vi "PH_BL-Master.set Instance remote controlled.vi"(0 "i ref in":refnum<vi>, 2 "Remote Controlled (false)":bool, 3 "Instance Name":string="N/A", 5 "error in":errorcluster) -> (14 "i ref out":refnum<vi>, 19 "error out":errorcluster)   [LabVIEW 2014, in "PH_BL-Master.lvlib"]
doc: "This VI checks the class of the instance and sets - if available - the instance remote controlled or releases this feature."
uses:
  PH_BL-Master.lvlib
  CSCore/CSSystem/CSSystemLib/CSSystemLib.lvlib
  PH_Sixpack_Switch/PH_Sixpack_Switch.lvlib
  PH_Switch/PH_Switch.lvlib
  PH_VacuumControl/PH_VacuumControl.lvlib
  PH_Common/PH_Common.lvlib
  PH_BlackBox/PH_BlackBox.lvlib
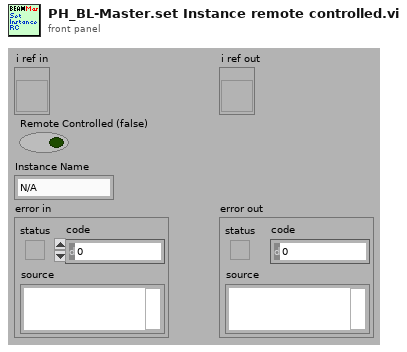
[diagram p1: front panel]
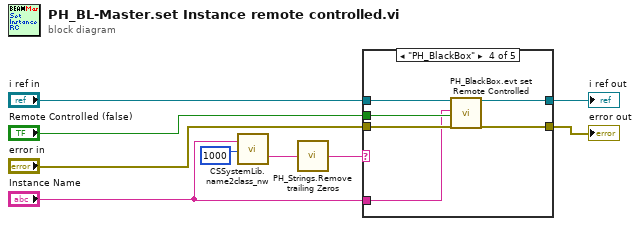
[diagram p0: block diagram]
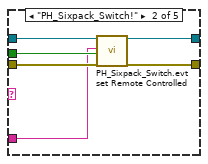
[diagram p3: hidden frame]
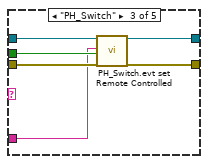
[diagram p4: hidden frame]
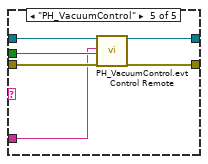
[diagram p5: hidden frame]
diagram:
  n1 = call "CSSystemLib.name2class_nw.vi"("name"="Instance Name", "timeout [ms] (10000)"=u32 1000) -> ("classID"=w2:string)  [unwired: 15 in, 2 out]
  n2 = call "PH_Strings.Remove trailing Zeros.vi"("Input String"=w2) -> ("Output String"=w1:string)
  n3 = case shown="\"PH_BlackBox\"" w1 {
    tunnel: "i ref in" -> [w11 w17 w23 w29 w35]
    tunnel: [w11 w16 w22 w28 w34] -> w5
    tunnel: "error in" -> [w10 w15 w21 w27 w33]
    tunnel: [w10 w14 w20 w26 w32] -> w7
    tunnel: "Remote Controlled (false)" -> [_ w13 w19 w25 w31]
    tunnel: "Instance Name" -> [_ w12 w18 w24 w30]
    frame Default {
    }
    frame "PH_Sixpack_Switch!" {
      n4 = call "PH_Sixpack_Switch.evt set Remote Controlled.vi"("i ref in"=w17, "Instance"=w12, "Remote Controlled"=w13, "error in (no error)"=w15) -> ("i ref out"=w16:refnum<vi>, "error out"=w14:errorcluster)  [unwired: 14 in]
    }
    frame "PH_Switch" {
      n5 = call "PH_Switch.evt set Remote Controlled.vi"("i ref in"=w23, "Instance"=w18, "Remote Controlled"=w19, "error in (no error)"=w21) -> ("i ref out"=w22:refnum<vi>, "error out"=w20:errorcluster)  [unwired: 14 in]
    }
    frame "PH_BlackBox" {
      n6 = call "PH_BlackBox.evt set Remote Controlled.vi"("i ref in"=w29, "Instance"=w24, "Remote Controlled?"=w25, "error in (no error)"=w27) -> ("i ref out"=w28:refnum<vi>, "error out"=w26:errorcluster)  [unwired: 14 in]
    }
    frame "PH_VacuumControl" {
      n7 = call "PH_VacuumControl.evt Control Remote.vi"("i ref in"=w35, "Instance"=w30, "Control Remote?"=w31, "error in (no error)"=w33) -> ("i ref out"=w34:refnum<vi>, "error out"=w32:errorcluster)  [unwired: 14 in]
    }
  }
  "error out" <- w7
  "i ref out" <- w5
